vi "Main Page.vi"(8 "error in":errorcluster, 11 "Node Ptr":T2 format="%.0x") -> (0 "error out":errorcluster)   [LabVIEW 2020, in "Ballard MIL-STD-1553 System Explorer.lvlib" / "Implementation.lvlib"]
uses:
  Implementation.lvlib
  <vilib>/NI VeriStand/Custom Device API/Custom Device Item Ref.ctl
  Shared/Initialization Method.ctl
  <vilib>/NI VeriStand/Custom Device API/Custom Device API.lvlib
  Scripting/Ballard MIL-STD-1553 Scripting.lvlib
panel:
  in  "Decimation":i32=1 min=0 step=1
  in  "Async Rx Execution":bool
  in  "core number":i32 caption="Core Number" min=0 step=1
  in  "number":i32=1 caption="PXI Slot Number" min=0 step=1
  in  "initialization method":T1 caption="Initialization Method"
  out "Version":string
  in  "SHDocVw.IWebBrowser":refnum<k7>(container)
  in  "General Header":cluster{"Section Name":string}={"Section Name"="Ballard MIL-STD-1553 - Main"}
  in  "Description":string
  in  "Name":string
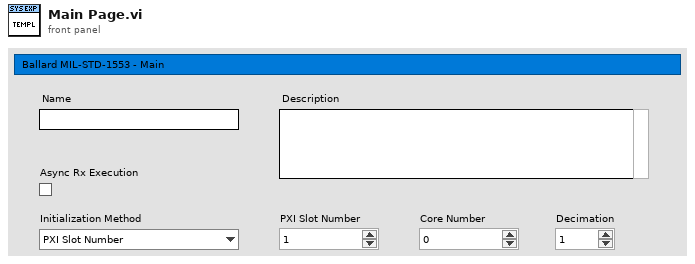
[diagram p1: front panel]
types:
  T1 = typedef "Initialization Method.ctl" = enum16{"PXI Slot Number", "Card Number"}
  T2 = typedef "Custom Device API.lvlib/Custom Device Item Ref.ctl" = u64
  T3 = typedef "Device Parameters.ctl" = cluster{"initialization method":T1, "card number":i32, "PXI slot number":i32, "core number":i32}
  T4 = typedef "Custom Device API.lvlib/Custom Device Item Info.ctl" = cluster{"Name":string, "Is Channel":bool, "GUID":string, "Is Waveform":bool}
  T5 = typedef "Custom Device API.lvlib/Custom Device Commands.ctl" = enum16{"Default", "Item renamed", "Shutdown", "Dynamic button pressed"}
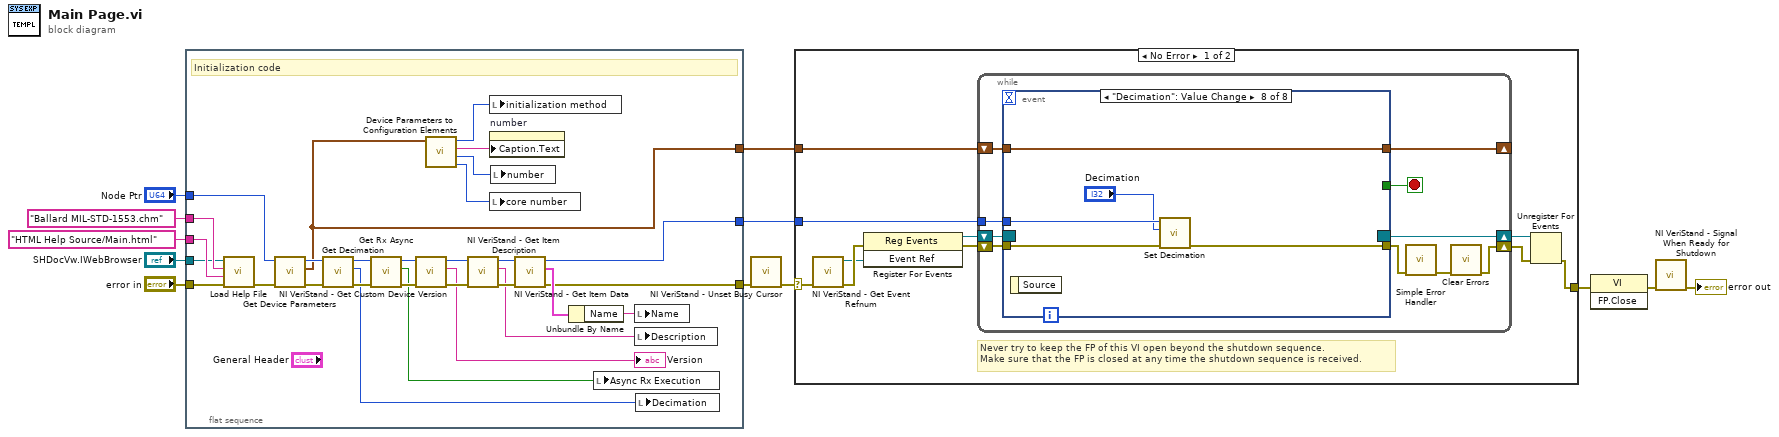
[diagram p0: block diagram]
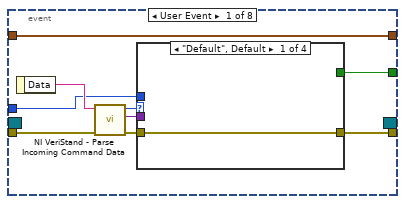
[diagram p2: hidden frame]
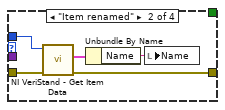
[diagram p3: hidden frame]
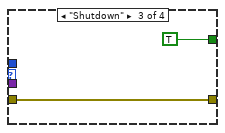
[diagram p4: hidden frame]
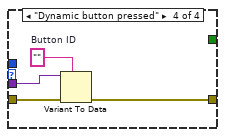
[diagram p5: hidden frame]
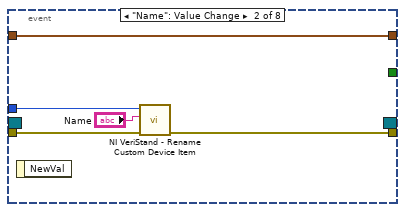
[diagram p6: hidden frame]
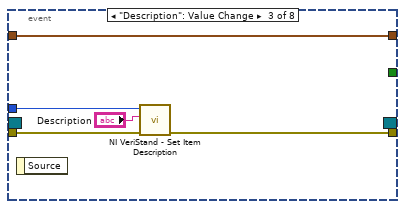
[diagram p7: hidden frame]
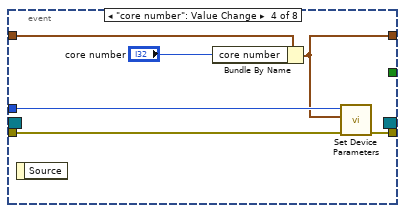
[diagram p8: hidden frame]
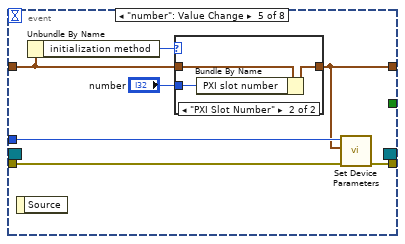
[diagram p9: hidden frame]
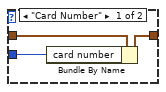
[diagram p10: hidden frame]
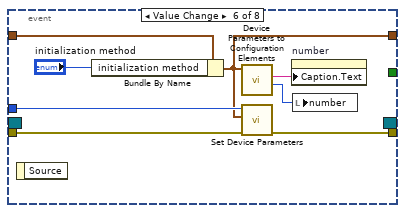
[diagram p11: hidden frame]
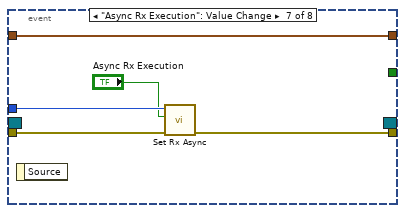
[diagram p12: hidden frame]
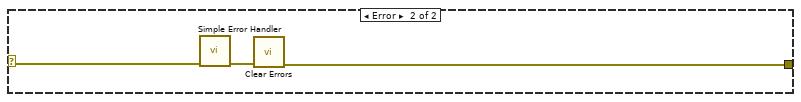
[diagram p13: hidden frame]
diagram:
  n1 = flat-sequence "Initialization code" {
    tunnel: "error in" -> [w33]
    tunnel: "Node Ptr" -> [w28]
    tunnel: [w24] -> w8
    tunnel: [w25] -> w5
    tunnel: "SHDocVw.IWebBrowser" -> [w30]
    tunnel: "HTML Help Source/Main.html" ("HTML File") -> [w31]
    tunnel: "Ballard MIL-STD-1553.chm" ("CD_CHM_FileName") -> [w32]
    tunnel: [w20] -> w1
    frame #0 {
      # "Initialization code"
      n2 = call "Load Help File.vi"("error in (no error)"=w33, "HTML File to Load"=w31, "Main CHM File"=w32, "Browser"=w30) -> ("error out"=w27:errorcluster)  [unwired: 7 in]
      n3 = call "Get Device Parameters.vi"("error in"=w27, "Ballard MIL-STD 1553 custom device in"=w28) -> ("error out"=w15:errorcluster, "device parameters"=w20:T3, "Ballard MIL-STD 1553 custom device out"=w26:T2)  [unwired: 7 in]
      n4 = call "Get Decimation.vi"("error in"=w15, "Ballard MIL-STD 1553 custom device in"=w26) -> ("error out"=w14:errorcluster, "decimation"=w13:i32, "Ballard MIL-STD 1553 custom device out"=w16:T2)  [unwired: 7 in]
      n5 = call "Get Rx Async.vi"("error in"=w14, "Ballard MIL-STD 1553 custom device in"=w16) -> ("error out"=w18:errorcluster, "Rx Async?"=w17:bool, "Ballard MIL-STD 1553 custom device out"=w19:T2)  [unwired: 7 in]
      n6 = call <vilib>:"NI VeriStand - Get Custom Device Version.vi"("error in (no error)"=w18, "Device Ref in"=w19) -> ("error out"=w38:errorcluster, "Value"=→"Version":string, "Device Ref out"=w37:T2)  [unwired: 7 in]
      n7 = call "Device Parameters to Configuration Elements.vi"("device parameters"=w20) -> ("core number"=w21:i32, "number"=w22:i32, "number caption"=w23:string, "initialization method"=w29:T1)  [unwired: 7 in]
      n8 = call <vilib>:"NI VeriStand - Get Item Description.vi"("error in (no error)"=w38, "Item Ref in"=w37) -> ("error out"=w40:errorcluster, "Description"=w34:string, "Item Ref out"=w41:T2)  [unwired: 7 out]
      n9 = local write "initialization method"(w29) -> ()
      n10 = property on="number" class="DigNum (strict)"("Caption.Text"=w23) -> ()  [unwired: 2 in, 2 out]
      n11 = local write "core number"(w21) -> ()
      n12 = local write "number"(w22) -> ()
      n13 = call <vilib>:"NI VeriStand - Get Item Data.vi"("error in (no error)"=w40, "Item Ref in"=w41) -> ("error out"=w24:errorcluster, "Item Info"=w39:T4, "Item Ref out"=w25:T2)  [unwired: 7 out]
      n14 = Unbundle By Name(w39) -> ("Name"=w35:string)
      n15 = local write "Async Rx Execution"(w17) -> ()
      n16 = local write "Name"(w35) -> ()
      n17 = local write "Description"(w34) -> ()
      n18 = local write "Decimation"(w13) -> ()
    }
  }
  n19 = call <vilib>:"NI VeriStand - Unset Busy Cursor.vi"("error in (no error)"=w8) -> ("error out"=w7:errorcluster)  [unwired: 10 out]
  n20 = case shown="No Error" w7 {
    selector: w7 -> [w43 w132]
    tunnel: [w48 w130] -> w12
    tunnel: w5 -> [w44 _]
    tunnel: w1 -> [w42 _]
    frame No Error {
      # "Never try to keep the FP of this VI open beyond the shutdown sequence.\nMake sure that the FP is closed at any time the shutdown sequence is received."
      n21 = call <vilib>:"NI VeriStand - Get Event Refnum.vi"("error in (no error)"=w43) -> ("error out"=w51:errorcluster, "Event Ref"=w47:refnum<user-event>)  [unwired: 9 out]
      n22 = register-events(error in=w51, w47) -> (reference out=w45:refnum<event-registration>, error out=w46:errorcluster)  [unwired: 1 in]
      n23 = while {
        tunnel: w44 -> [w57]
        shift-right: [w54] -> w49
        shift-left: w46 -> [w60]
        shift-right: [w61] -> w50
        shift-left: w45 -> [w59]
        shift-right: [w52] -> _
        shift-left: w42 -> [w53]
        stop <- w58 stop-if-true
        n24 = event shown="[7] \"Decimation\": Value Change" {
          selector: w59 -> [_ _ _ _ _ _ _ _]
          dyn-events: [_ _ _ _ _ _ _ _] -> w61
          timeout: _ -> [_ _ _ _ _ _ _ _]
          tunnel: w60 -> [w70 w87 w91 w94 w102 w113 w123 w128]
          tunnel: [w66 _ _ _ _ _ _ _] -> w58
          tunnel: [w65 w86 w90 w95 w101 w112 w120 w126] -> w56
          tunnel: w57 -> [w62 w85 w92 w96 w100 w115 w122 w127]
          tunnel: w53 -> [w63 w83 w88 w98 w104 w117 w124 w129]
          tunnel: [w63 w83 w88 w93 w99 w114 w124 w129] -> w52
          event User Event {
            n25 = event-data() -> ("Data"=w69:string)  [unwired: 1 out]
            n26 = call <vilib>:"NI VeriStand - Parse Incoming Command Data.vi"("error in (no error)"=w70, "Incoming data"=w69) -> ("error out"=w68:errorcluster, "Outgoing data"=w64:variant, "Action"=w67:T5)  [unwired: 7 out]
            n27 = case shown="\"Default\", Default" w67 {
              tunnel: w68 -> [w71 w76 w77 w82]
              tunnel: [_ _ TRUE _] -> w66
              tunnel: [w71 w73 w77 w79] -> w65
              tunnel: w62 -> [_ w75 _ _]
              tunnel: w64 -> [_ _ _ w81]
              frame "Default", Default {
              }
              frame "Item renamed" {
                n28 = call <vilib>:"NI VeriStand - Get Item Data.vi"("error in (no error)"=w76, "Item Ref in"=w75) -> ("error out"=w73:errorcluster, "Item Info"=w74:T4)  [unwired: 8 out]
                n29 = Unbundle By Name(w74) -> ("Name"=w72:string)
                n30 = local write "Name"(w72) -> ()
              }
              frame "Shutdown" {
              }
              frame "Dynamic button pressed" {
                w80 = ""  # Button ID
                n31 = Variant To Data(error in=w82, type=w80, Variant=w81) -> (error out=w79:errorcluster)  [unwired: 1 out]
              }
            }
          }
          event "Name": Value Change {
            n32 = event-data() -> ()  [unwired: 2 out]
            n33 = call <vilib>:"NI VeriStand - Rename Custom Device Item.vi"("error in (no error)"=w87, "New Name"="Name", "Item Ref in"=w85) -> ("error out"=w86:errorcluster)  [unwired: 1 in, 7 out]
          }
          event "Description": Value Change {
            n34 = event-data() -> ()  [unwired: 2 out]
            n35 = call <vilib>:"NI VeriStand - Set Item Description.vi"("error in (no error)"=w91, "Description"="Description", "Item Ref in"=w92) -> ("error out"=w90:errorcluster)  [unwired: 8 out]
          }
          event "core number": Value Change {
            n36 = event-data() -> ()  [unwired: 2 out]
            n37 = Bundle By Name(cluster=w98, "core number"="core number") -> (w93:T3)
            n38 = call "Set Device Parameters.vi"("error in"=w94, "device parameters"=w93, "Ballard MIL-STD 1553 custom device in"=w96) -> ("error out"=w95:errorcluster)  [unwired: 7 in, 1 out]
          }
          event "number": Value Change {
            n39 = event-data() -> ()  [unwired: 2 out]
            n40 = Unbundle By Name(w104) -> ("initialization method"=w105:T1)
            n41 = case shown="\"PXI Slot Number\"" w105 {
              tunnel: w104 -> [w108 w111]
              tunnel: "number" -> [w107 w110]
              tunnel: [w106 w109] -> w99
              frame "Card Number" {
                n42 = Bundle By Name(cluster=w108, "card number"=w107) -> (w106:T3)
              }
              frame "PXI Slot Number" {
                n43 = Bundle By Name(cluster=w111, "PXI slot number"=w110) -> (w109:T3)
              }
            }
            n44 = call "Set Device Parameters.vi"("error in"=w102, "device parameters"=w99, "Ballard MIL-STD 1553 custom device in"=w100) -> ("error out"=w101:errorcluster)  [unwired: 7 in, 1 out]
          }
          event Value Change {
            n45 = event-data() -> ()  [unwired: 2 out]
            n46 = Bundle By Name(cluster=w117, "initialization method"="initialization method") -> (w114:T3)
            n47 = call "Device Parameters to Configuration Elements.vi"("device parameters"=w114) -> ("number"=w118:i32, "number caption"=w119:string)  [unwired: 7 in, 2 out]
            n48 = call "Set Device Parameters.vi"("error in"=w113, "device parameters"=w114, "Ballard MIL-STD 1553 custom device in"=w115) -> ("error out"=w112:errorcluster)  [unwired: 7 in, 1 out]
            n49 = property on="number" class="DigNum (strict)"("Caption.Text"=w119) -> ()  [unwired: 2 in, 2 out]
            n50 = local write "number"(w118) -> ()
          }
          event "Async Rx Execution": Value Change {
            n51 = event-data() -> ()  [unwired: 2 out]
            n52 = call "Set Rx Async.vi"("error in"=w123, "Rx Async?"="Async Rx Execution", "Ballard MIL-STD 1553 custom device in"=w122) -> ("error out"=w120:errorcluster)  [unwired: 7 in, 1 out]
          }
          event "Decimation": Value Change {
            n53 = event-data() -> ()  [unwired: 2 out]
            n54 = call "Set Decimation.vi"("error in"=w128, "decimation"="Decimation", "Ballard MIL-STD 1553 custom device in"=w127) -> ("error out"=w126:errorcluster)  [unwired: 7 in, 1 out]
          }
        }
        n55 = call <vilib>:"Simple Error Handler.vi"("error in (no error)"=w56) -> ("error out"=w55:errorcluster)  [unwired: 1 in, 7 out]
        n56 = call <vilib>:"Clear Errors.vi"("error in (no error)"=w55) -> ("error out"=w54:errorcluster)  [unwired: 1 in, 5 out]
      }
      n57 = Unregister For Events(event registration refnum=w50, error in=w49) -> (error out=w48:errorcluster)
    }
    frame Error {
      n58 = call <vilib>:"Simple Error Handler.vi"("error in (no error)"=w132) -> ("error out"=w131:errorcluster)  [unwired: 1 in, 7 out]
      n59 = call <vilib>:"Clear Errors.vi"("error in (no error)"=w131) -> ("error out"=w130:errorcluster)  [unwired: 1 in, 5 out]
    }
  }
  n60 = invoke class="VI" method="FP.Close"(error in=w12) -> (error out=w11:errorcluster)  [unwired: 2 in, 2 out]
  n61 = call <vilib>:"NI VeriStand - Signal When Ready for Shutdown.vi"("error in (no error)"=w11) -> ("error out"=→"error out":errorcluster)  [unwired: 10 out]
